vi "Does_file_exist_(simple).vi"(1 "Pathname":path) -> (0 "exists?":bool)   [LabVIEW 2010]
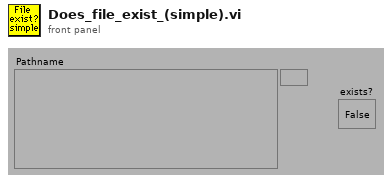
[diagram p1: front panel]
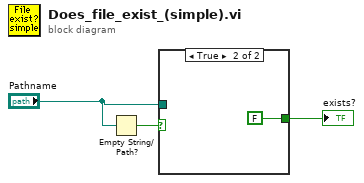
[diagram p0: block diagram]
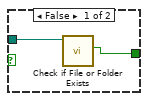
[diagram p2: hidden frame]
diagram:
  n1 = Empty String/Path?(string/path="Pathname") -> (empty?=w2:bool)
  n2 = case shown="True" w2 {
    tunnel: "Pathname" -> [w5 _]
    tunnel: [w4 FALSE ("file or folder exists?")] -> w1
    frame False {
      n3 = call <vilib>:"Check if File or Folder Exists.vi"("path"=w5) -> ("file or folder exists?"=w4:bool)  [unwired: 1 in, 9 out]
    }
    frame True {
    }
  }
  "exists?" <- w1
